vi "stop_watch_w_feedback_node2.vi"(10 "Command":enum16{"Elapsed Time", "Reset"}(ring)) -> (2 "Elapsed Time":dbl)   [LabVIEW 2015]
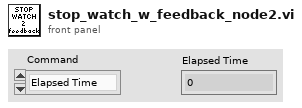
[diagram p1: front panel]
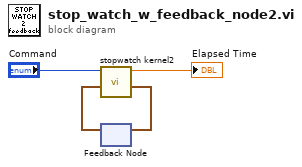
[diagram p0: block diagram]
diagram:
  n1 = feedback #1() -> (w1:cluster{"Timestamp":dbl, "Elapsed Time":dbl})  [unwired: 1 in]
  n2 = call "stopwatch kernel2.vi"("State variables in"=w1, "Command"="Command") -> ("State variables out"=w2:cluster{"Timestamp":dbl, "Elapsed Time":dbl}, "Elapsed Time"=→"Elapsed Time":dbl)  [unwired: 8 in]
  n3 = feedback-in #1(w2) -> ()
